vi "error.handler.vi"(8 "error in (no error)":errorcluster, 11 "ComicVine_manager in":refnum<class "CV_downloader.lvclass">) -> (0 "error out":errorcluster, 3 "ComicVine_manager out":refnum<class "CV_downloader.lvclass">)   [LabVIEW 2024, in "CV_downloader.lvclass"]
uses:
  CV_downloader.lvclass
  states--enum.ctl
  CV_downloader.lvclass/CV_downloader.ctl
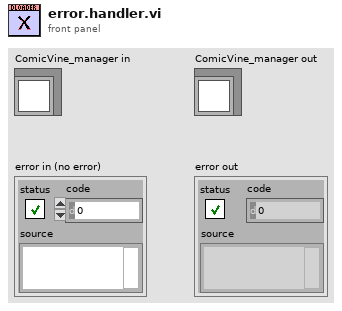
[diagram p1: front panel]
types:
  T1 = typedef "CV_downloader.lvclass/states--enum.ctl" = enum16{"start", "running", "start timer", "update file", "set directories", "wait", "shutdown"}
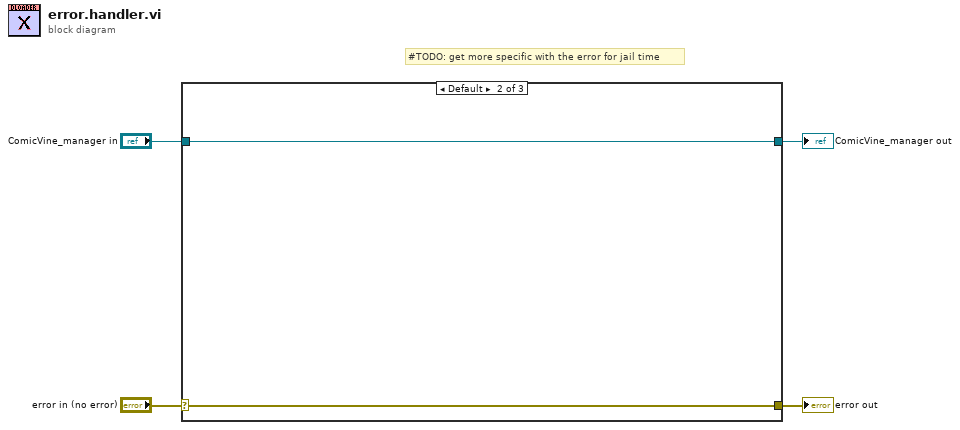
[diagram p0: block diagram]
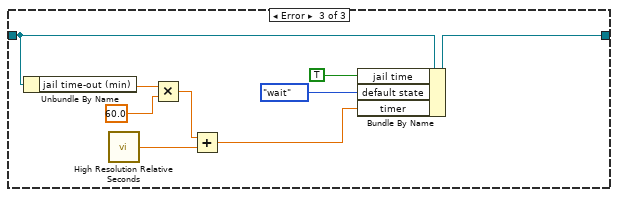
[diagram p3: hidden frame]
diagram:
  # "#TODO: get more specific with the error for jail time"
  n1 = case shown="Default" "error in (no error)" {
    selector: "error in (no error)" -> [w5 w8 _]
    tunnel: [w5 w8 _] -> w3
    tunnel: [w6 w7 w16] -> w1
    tunnel: "ComicVine_manager in" -> [w6 w7 w13]
    frame No Error {
    }
    frame Default {
    }
    frame Error {
      n2 = Unbundle By Name(w13) -> ("jail time-out (min)"=w12:dbl)
      n3 = call <vilib>:"High Resolution Relative Seconds.vi"() -> ("relative seconds"=w14:dbl)
      n4 = Multiply(x=w12, y=60.0) -> (x*y=w10:dbl)
      n5 = Add(x=w10, y=w14) -> (x+y=w9:dbl)
      n6 = Bundle By Name(cluster=w13, "jail time"=TRUE, "default state"=states--enum."wait", "timer"=w9) -> (w16:refnum<class "CV_downloader.lvclass">)
    }
  }
  "error out" <- w3
  "ComicVine_manager out" <- w1
